vi "Insight_SweepStart_Trigger.vi"(8 "error in (no error)":errorcluster, 9 "Mode (Read / Write)":enum8{"Write", "Read"}(ring), 10 "Sweep Start Trigger Edge":T1=enum."BOTH", 11 "telnet connection":T2) -> (0 "error out":errorcluster, 1 "Sweep Start Trigger Edge?":T1=enum."BOTH", 2 "response data":string, 3 "telnet  connection out":T2)   [LabVIEW 2011]
doc: "Insight Photonic Solutions\n\nThis VI sets or queries what edge of the Sweep Start Trigger signal corresponds with the start of the sweep of the laser. Options are Rising, Falling or Both.\n\nver 1.0 - original release\nver 1.0.1 - fixed parser implementation\nver 3.3 - modified to support earlier versions of this command (v3.2 and earlier), and current response format (3.3 and later)"
uses:
  Telnet Session.ctl
  Start_Sweep_Trigger.ctl
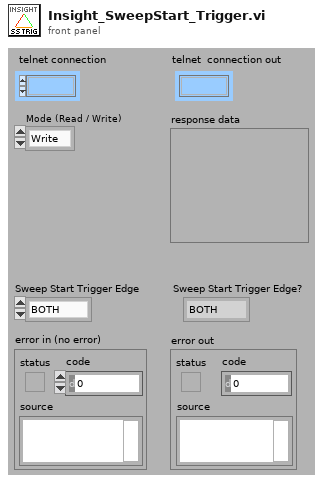
[diagram p1: front panel]
types:
  T1 = typedef "Start_Sweep_Trigger.ctl" = enum16{"RISing", "FALLing", "BOTH"}
  T2 = typedef "Telnet Session.ctl" = refnum<k1>
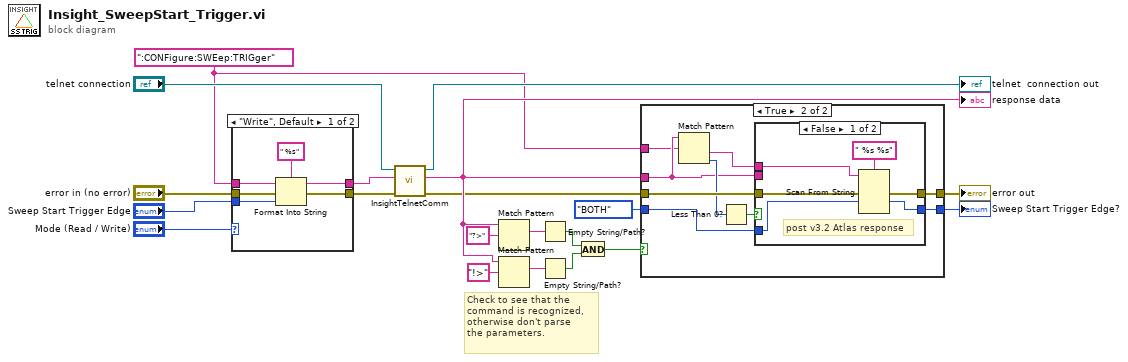
[diagram p0: block diagram]
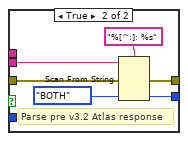
[diagram p3: hidden frame]
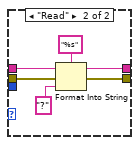
[diagram p4: hidden frame]
diagram:
  w2 = ":CONFigure:SWEep:TRIGger" ("String")
  # "Check to see that the \ncommand is recognized,\notherwise don't parse \nthe parameters."
  n1 = case shown="\"Write\", Default" "Mode (Read / Write)" {
    tunnel: [w26 w28] -> w18
    tunnel: "error in (no error)" -> [w25 w27]
    tunnel: w2 -> [w24 w30]
    tunnel: "Sweep Start Trigger Edge" -> [w23 _]
    tunnel: [w21 w29] -> w17
    frame "Write", Default {
      n2 = Format Into String(format string=" %s", initial string=w24, error in=w25, w23) -> (resulting string=w21:string, error out=w26:errorcluster)
    }
    frame "Read" {
      n3 = Format Into String(format string="%s", initial string=w30, error in=w27, "?" ("input 1")) -> (resulting string=w29:string, error out=w28:errorcluster)
    }
  }
  n4 = call "InsightTelnetComm.vi"("error in"=w18, "write buffer (\"\")"=w17, "telnet connection"="telnet connection") -> ("error out"=w5:errorcluster, "response data"=w6:string, "telnet  connection out"=→"telnet  connection out":T2)  [unwired: 4 in]
  "response data" <- w6
  n5 = Match Pattern(string=w6, regular expression="?>") -> (match substring=w9:string)  [unwired: 1 in, 3 out]
  n6 = Match Pattern(string=w6, regular expression="!>") -> (match substring=w10:string)  [unwired: 1 in, 3 out]
  n7 = Empty String/Path?(string/path=w9) -> (empty?=w12:bool)
  n8 = Empty String/Path?(string/path=w10) -> (empty?=w13:bool)
  n9 = And(x=w12, y=w13) -> (x .and. y?=w7:bool)
  n10 = case shown="True" w7 {
    tunnel: [w34 w41] -> w4
    tunnel: w5 -> [w34 w40]
    tunnel: w6 -> [_ w37]
    tunnel: [w33 w42] -> w1
    tunnel: w2 -> [_ w36]
    tunnel: Start_Sweep_Trigger."BOTH" ("Sweep Start Trigger Edge") -> [w33 w35]
    frame False {
    }
    frame True {
      n11 = Match Pattern(string=w37, regular expression=w36) -> (after substring=w38:string, offset past match=w39:i32)  [unwired: 1 in, 2 out]
      n12 = Less Than 0?(x=w39) -> (x < 0?=w43:bool)
      n13 = case shown="False" w43 {
        tunnel: w38 -> [w48 _]
        tunnel: w37 -> [_ w54]
        tunnel: [w49 w55] -> w41
        tunnel: [w46 w52] -> w42
        tunnel: w40 -> [w45 w51]
        tunnel: w35 -> [w44 _]
        frame False {
          # "post v3.2 Atlas response"
          n14 = Scan From String(format string=" %s %s" ("f"), input string=w48, error in=w45, default 1=w44) -> (error out=w49:errorcluster, output 1=w46:T1)  [unwired: 3 in, 2 out]
        }
        frame True {
          # "Parse pre v3.2 Atlas response"
          n15 = Scan From String(format string="%[^:]: %s", input string=w54, error in=w51, default 2=enum16{"RISING", "FALLING", "BOTH"}."BOTH") -> (error out=w55:errorcluster, output 2=w52:enum16{"RISING", "FALLING", "BOTH"})  [unwired: 3 in, 2 out]
        }
      }
    }
  }
  "error out" <- w4
  "Sweep Start Trigger Edge?" <- w1
